vi "MotorRun.vi"() -> ()   [LabVIEW 2011]
uses:
  API/API DYM.lvlib
panel:
  out "motor statue array output":i32[](array[numeric])
  in  "获取电机运行状态按钮":bool
  in  "SetSpeedStepNum":i32
  in  "SetSpeedmotorNum":i32
  in  "设定电机速度按钮":bool
  in  "电机复位编号":i32
  in  "电机复位按钮":bool
  in  "停止编号":i32
  in  "电机停止按钮":bool
  in  "stepNum6":i32
  in  "direction6":i32
  in  "motorNum6":i32
  in  "stepNum5":i32
  in  "direction5":i32
  in  "motorNum5":i32
  in  "stepNum4":i32
  in  "direction4":i32
  in  "motorNum4":i32
  in  "stepNum3":i32
  in  "direction3":i32
  in  "motorNum3":i32
  in  "六号电机驱动按钮":bool
  in  "五号电机驱动按钮":bool
  in  "四号电机驱动按钮":bool
  in  "三号电机驱动按钮":bool
  in  "进料电机停止按钮":bool
  in  "进料电机运行按钮":bool
  out "布尔":bool
  in  "启动按钮":bool
  in  "退出按钮":bool
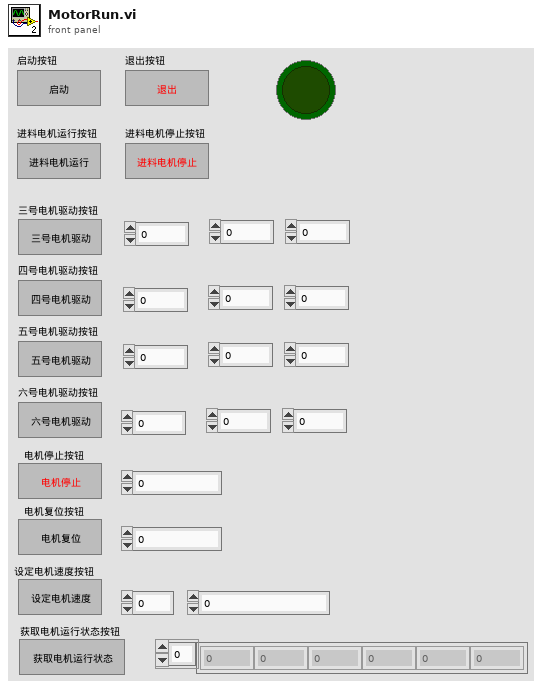
[diagram p1: front panel]
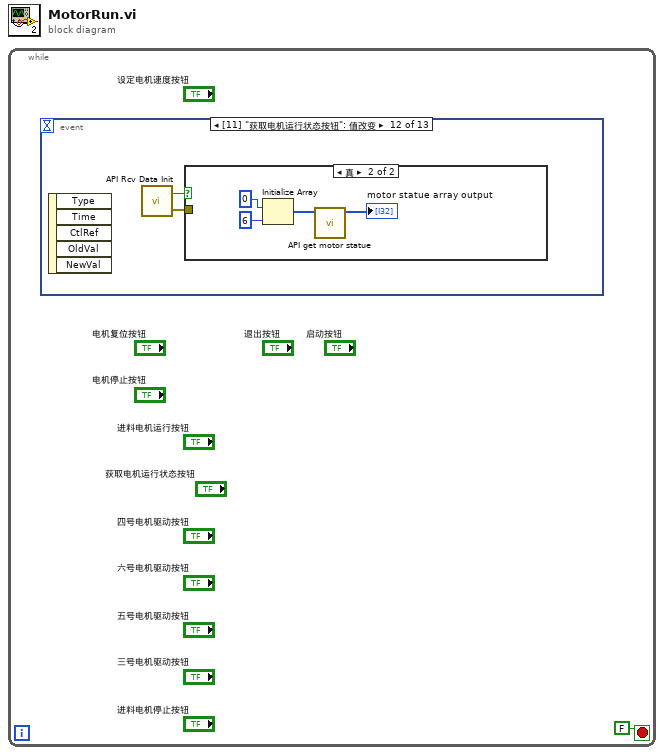
[diagram p0: block diagram]
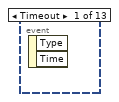
[diagram p2: hidden frame]
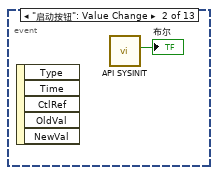
[diagram p3: hidden frame]
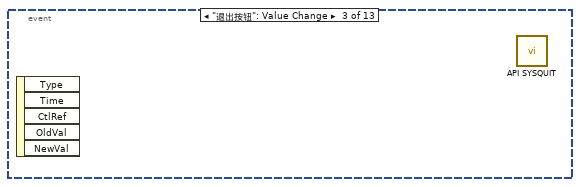
[diagram p4: hidden frame]
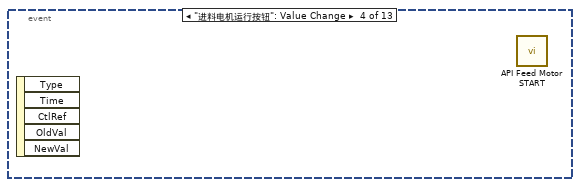
[diagram p5: hidden frame]
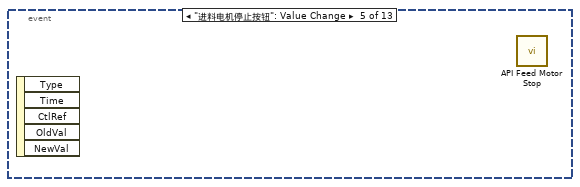
[diagram p6: hidden frame]
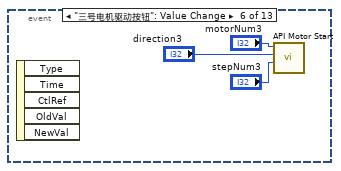
[diagram p7: hidden frame]
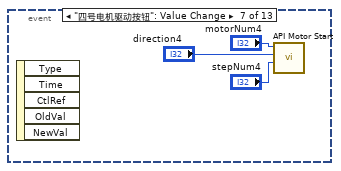
[diagram p8: hidden frame]
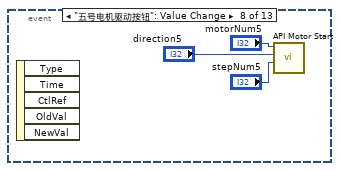
[diagram p9: hidden frame]
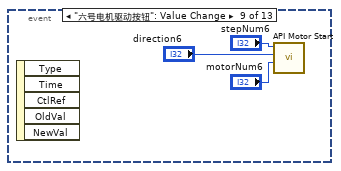
[diagram p10: hidden frame]
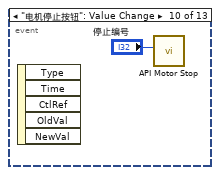
[diagram p11: hidden frame]
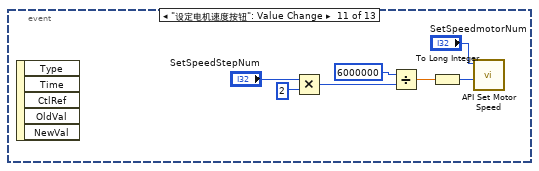
[diagram p12: hidden frame]
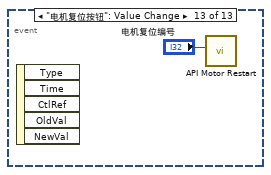
[diagram p14: hidden frame]
diagram:
  n1 = while {
    stop <- FALSE stop-if-true
    n2 = event shown="[11] \"获取电机运行状态按钮\": 值改变" {
      selector: _ -> [_ _ _ _ _ _ _ _ _ _ _ _ _]
      dyn-events: _ -> [_ _ _ _ _ _ _ _ _ _ _ _ _]
      timeout: _ -> [_ _ _ _ _ _ _ _ _ _ _ _ _]
      event Timeout {
        n3 = event-data() -> ()  [unwired: 1 in, 2 out]
      }
      event "启动按钮": Value Change {
        n4 = event-data() -> ()  [unwired: 1 in, 5 out]
        n5 = call "API SYSINIT.vi"() -> ("SYSINIT return value"=→"布尔":bool)  [unwired: 11 in]
      }
      event "退出按钮": Value Change {
        n6 = event-data() -> ()  [unwired: 1 in, 5 out]
        n7 = call "API SYSQUIT.vi"() -> ()  [unwired: 12 in]
      }
      event "进料电机运行按钮": Value Change {
        n8 = event-data() -> ()  [unwired: 1 in, 5 out]
        n9 = call "API Feed Motor START.vi"() -> ()  [unwired: 11 in, 1 out]
      }
      event "进料电机停止按钮": Value Change {
        n10 = event-data() -> ()  [unwired: 1 in, 5 out]
        n11 = call "API Feed Motor Stop.vi"() -> ()  [unwired: 11 in, 1 out]
      }
      event "三号电机驱动按钮": Value Change {
        n12 = event-data() -> ()  [unwired: 1 in, 5 out]
        n13 = call "API Motor Start.vi"("stepNum"="stepNum3", "direction"="direction3", "motorNum"="motorNum3") -> ()  [unwired: 8 in, 1 out]
      }
      event "四号电机驱动按钮": Value Change {
        n14 = event-data() -> ()  [unwired: 1 in, 5 out]
        n15 = call "API Motor Start.vi"("stepNum"="stepNum4", "direction"="direction4", "motorNum"="motorNum4") -> ()  [unwired: 8 in, 1 out]
      }
      event "五号电机驱动按钮": Value Change {
        n16 = event-data() -> ()  [unwired: 1 in, 5 out]
        n17 = call "API Motor Start.vi"("stepNum"="stepNum5", "direction"="direction5", "motorNum"="motorNum5") -> ()  [unwired: 8 in, 1 out]
      }
      event "六号电机驱动按钮": Value Change {
        n18 = event-data() -> ()  [unwired: 1 in, 5 out]
        n19 = call "API Motor Start.vi"("stepNum"="motorNum6", "direction"="direction6", "motorNum"="stepNum6") -> ()  [unwired: 8 in, 1 out]
      }
      event "电机停止按钮": Value Change {
        n20 = event-data() -> ()  [unwired: 1 in, 5 out]
        n21 = call "API Motor Stop.vi"("motorNum"="停止编号") -> ()  [unwired: 10 in, 1 out]
      }
      event "设定电机速度按钮": Value Change {
        n22 = event-data() -> ()  [unwired: 1 in, 5 out]
        n23 = Multiply(x="SetSpeedStepNum", y=2) -> (x*y=w19:i32)
        n24 = Divide(x=6000000, y=w19) -> (x/y=w17:dbl)
        n25 = To Long Integer(number=w17) -> (32bit integer=w16:i32)
        n26 = call "API Set Motor Speed.vi"("motorSpeed"=w16, "motorNum"="SetSpeedmotorNum") -> ()  [unwired: 9 in, 1 out]
      }
      event "获取电机运行状态按钮": Value Change {
        n27 = event-data() -> ()  [unwired: 1 in, 5 out]
        n28 = call "API Rcv Data Init.vi"() -> ("错误输出"=w23:errorcluster, "RTV"=w24:bool)  [unwired: 2 in]
        n29 = case shown="真" w24 {
          tunnel: w23 -> [_ _]
          frame False {
          }
          frame True {
            n30 = Initialize Array(0 ("元素"), 6 ("维数大小")) -> (w26:i32[])
            n31 = call "API get motor statue.vi"("motor statue array input"=w26) -> ("motor statue array output"=→"motor statue array output":i32[])  [unwired: 9 in, 1 out]
          }
        }
      }
      event "电机复位按钮": Value Change {
        n32 = event-data() -> ()  [unwired: 1 in, 5 out]
        n33 = call "API Motor Restart.vi"("motorNum"="电机复位编号") -> ()  [unwired: 10 in, 1 out]
      }
    }
  }
